vi "sv_Get Next Swept Frequency.vi"(7 "mode":enum16{"feedback", "deterministic"}(ring), 8 "error in (no error)":errorcluster, 11 "swept sine task in":T1={"source settings"={"AO task name"="", "source"=[]}, "stimulus settings"={"stimulus task name"="", "stimulus"=[]}, "response(s) settings"={"response task name"="", "response"=[]}, "measurement settings"={"AI sampling frequency"=51200.0, "AO sampling frequency"=1024.0, "AI block size"=1024, "AO block Size"=1024, "block duration [ms]"=1024.0, "number of AI channels"=0, "device propagation delay [samples]"=0.0, "total propagation time [samples]"=0.0, "DUT propagation time [ms]"=0.0}, "linlog"=enum."linear", "repeat"=enum."off", "frequency list"=[1.0], "amplitude list"=[1.0], "settling time"={"settle time"=0.015599999576807022, "settle cycles"=5}, "integration time"={"integration time"=0.015599999576807022, "integration cycles"=5}, "frequencies indices"={"AI freq index"=0, "AO freq index"=5}, "read marks"={"write index"=0, "read index"=0, "freq start index"=0, "freq stop index"=0, "# extracted"=0, "buffer type"=enum."Invalid buffer", "read/write indices"=[], "AO index"=0, "AI index"=0, "settled"=FALSE, "integration done"=FALSE}, "harmonic settings"={"maximum THD harmonic"=5, "harmonic mapping"=[1], "units"={"THD unit"=enum."%", "nth harmonic unit"=enum."%", "SINAD unit"=enum."dB", "THD+N unit"=enum."dB"}}, "auto resolution settings"={"auto max step"=512, "slow threshold db"=6.0, "fast threshold db"=1.0}, "auto level settings"={"auto level enable"=FALSE, "auto level channel"=6, "ideal ref"=1.0, "max level"=10.0, "ref upper deviation db"=3.0, "ref lower deviation db"=-3.0}, "offset"=1.0, "ramping rate"=0.0, "phase"=1.0, "initialize"=FALSE} {"phase" format="%.2f"; "response(s) settings"."response"."channel info"."pregain" format="%.2f"; "response(s) settings"."response"."channel info"."weighting filter" items=["Linear", "A-weighting", "B-weighting", "C-weighting", "ITU-R 468-4", "Dolby", "CCITT", "C-message", "Wb", "Wc", "Wd", "We", "Wf", "Wh", "Wj", "Wk", "Wm", "AES17 20 kHz lowpass", "AES17 40 kHz lowpass", "AES17 20 kHz highpass", "AES17 40 kHz highpass"]; "response(s) settings"."response"."channel info"."dB reference" format="%^.1e"; "response(s) settings"."response"."channel info"."engineering units" items=["custom..."=0, "V"=1, "A"=21, "C"=30, "pC"=31, "s"=32, "-"=29, "Pa"=2, "N"=20, "g"=3, "m/s^2"=4, "m/s"=5, "m"=6, "mm/s"=12, "mm"=13, "micron/s"=14, "micron"=15, "in/s^2"=7, "in/s"=8, "in"=9, "mil/s"=10, "mil"=11, "rad/s^2"=16, "rad/s"=17, "rad"=18, "deg/s^2"=26, "deg/s"=27, "deg"=28, "RPM"=22, "cycle/s^2"=23, "Hz"=24, "cycle"=25, "strain"=19]; "response(s) settings"."response"."channel info"."sensor sensitivity" format="%#_5f"; "stimulus settings"."stimulus"."channel info"."pregain" format="%.2f"; "stimulus settings"."stimulus"."channel info"."weighting filter" items=["Linear", "A-weighting", "B-weighting", "C-weighting", "ITU-R 468-4", "Dolby", "CCITT", "C-message", "Wb", "Wc", "Wd", "We", "Wf", "Wh", "Wj", "Wk", "Wm", "AES17 20 kHz lowpass", "AES17 40 kHz lowpass", "AES17 20 kHz highpass", "AES17 40 kHz highpass"]; "stimulus settings"."stimulus"."channel info"."dB reference" format="%^.1e"; "stimulus settings"."stimulus"."channel info"."engineering units" items=["custom..."=0, "V"=1, "A"=21, "C"=30, "pC"=31, "s"=32, "-"=29, "Pa"=2, "N"=20, "g"=3, "m/s^2"=4, "m/s"=5, "m"=6, "mm/s"=12, "mm"=13, "micron/s"=14, "micron"=15, "in/s^2"=7, "in/s"=8, "in"=9, "mil/s"=10, "mil"=11, "rad/s^2"=16, "rad/s"=17, "rad"=18, "deg/s^2"=26, "deg/s"=27, "deg"=28, "RPM"=22, "cycle/s^2"=23, "Hz"=24, "cycle"=25, "strain"=19]; "stimulus settings"."stimulus"."channel info"."sensor sensitivity" format="%#_5f"; "ramping rate" format="%.4f"; "offset" format="%.2f"; "auto level settings"."ref lower deviation db" format="%.4f"; "auto level settings"."ref upper deviation db" format="%.4f"; "auto level settings"."max level" format="%.4f"; "auto level settings"."ideal ref" format="%.4f"; "auto resolution settings"."fast threshold db" format="%.4f"; "auto resolution settings"."slow threshold db" format="%.4f"; "harmonic settings"."maximum THD harmonic" max=10 step=1; "integration time"."integration time" format="%.2p"; "settling time"."settle time" format="%.2p"; "amplitude list" format="%.2f"; "frequency list" format="%.2f"; "measurement settings"."DUT propagation time [ms]" format="%.2f"; "measurement settings"."AO sampling frequency" format="%.2f"; "measurement settings"."AI sampling frequency" format="%.2f"}) -> (0 "error out":errorcluster, 2 "stimulus":dbl[](array[numeric]) format="%.2f", 3 "swept sine task out":T1={"source settings"={"AO task name"="", "source"=[]}, "stimulus settings"={"stimulus task name"="", "stimulus"=[]}, "response(s) settings"={"response task name"="", "response"=[]}, "measurement settings"={"AI sampling frequency"=51200.0, "AO sampling frequency"=1024.0, "AI block size"=1024, "AO block Size"=1024, "block duration [ms]"=1024.0, "number of AI channels"=0, "device propagation delay [samples]"=0.0, "total propagation time [samples]"=0.0, "DUT propagation time [ms]"=0.0}, "linlog"=enum."linear", "repeat"=enum."off", "frequency list"=[1.0], "amplitude list"=[1.0], "settling time"={"settle time"=0.015599999576807022, "settle cycles"=5}, "integration time"={"integration time"=0.015599999576807022, "integration cycles"=5}, "frequencies indices"={"AI freq index"=0, "AO freq index"=5}, "read marks"={"write index"=0, "read index"=0, "freq start index"=0, "freq stop index"=0, "# extracted"=0, "buffer type"=enum."Invalid buffer", "read/write indices"=[], "AO index"=0, "AI index"=0, "settled"=FALSE, "integration done"=FALSE}, "harmonic settings"={"maximum THD harmonic"=5, "harmonic mapping"=[1], "units"={"THD unit"=enum."%", "nth harmonic unit"=enum."%", "SINAD unit"=enum."dB", "THD+N unit"=enum."dB"}}, "auto resolution settings"={"auto max step"=512, "slow threshold db"=6.0, "fast threshold db"=1.0}, "auto level settings"={"auto level enable"=FALSE, "auto level channel"=6, "ideal ref"=1.0, "max level"=10.0, "ref upper deviation db"=3.0, "ref lower deviation db"=-3.0}, "offset"=1.0, "ramping rate"=0.0, "phase"=1.0, "initialize"=FALSE} {"phase" format="%.2f"; "response(s) settings"."response"."channel info"."pregain" format="%.2f"; "response(s) settings"."response"."channel info"."weighting filter" items=["Linear", "A-weighting", "B-weighting", "C-weighting", "ITU-R 468-4", "Dolby", "CCITT", "C-message", "Wb", "Wc", "Wd", "We", "Wf", "Wh", "Wj", "Wk", "Wm", "AES17 20 kHz lowpass", "AES17 40 kHz lowpass", "AES17 20 kHz highpass", "AES17 40 kHz highpass"]; "response(s) settings"."response"."channel info"."dB reference" format="%^.1e"; "response(s) settings"."response"."channel info"."engineering units" items=["custom..."=0, "V"=1, "A"=21, "C"=30, "pC"=31, "s"=32, "-"=29, "Pa"=2, "N"=20, "g"=3, "m/s^2"=4, "m/s"=5, "m"=6, "mm/s"=12, "mm"=13, "micron/s"=14, "micron"=15, "in/s^2"=7, "in/s"=8, "in"=9, "mil/s"=10, "mil"=11, "rad/s^2"=16, "rad/s"=17, "rad"=18, "deg/s^2"=26, "deg/s"=27, "deg"=28, "RPM"=22, "cycle/s^2"=23, "Hz"=24, "cycle"=25, "strain"=19]; "response(s) settings"."response"."channel info"."sensor sensitivity" format="%#_5f"; "stimulus settings"."stimulus"."channel info"."pregain" format="%.2f"; "stimulus settings"."stimulus"."channel info"."weighting filter" items=["Linear", "A-weighting", "B-weighting", "C-weighting", "ITU-R 468-4", "Dolby", "CCITT", "C-message", "Wb", "Wc", "Wd", "We", "Wf", "Wh", "Wj", "Wk", "Wm", "AES17 20 kHz lowpass", "AES17 40 kHz lowpass", "AES17 20 kHz highpass", "AES17 40 kHz highpass"]; "stimulus settings"."stimulus"."channel info"."dB reference" format="%^.1e"; "stimulus settings"."stimulus"."channel info"."engineering units" items=["custom..."=0, "V"=1, "A"=21, "C"=30, "pC"=31, "s"=32, "-"=29, "Pa"=2, "N"=20, "g"=3, "m/s^2"=4, "m/s"=5, "m"=6, "mm/s"=12, "mm"=13, "micron/s"=14, "micron"=15, "in/s^2"=7, "in/s"=8, "in"=9, "mil/s"=10, "mil"=11, "rad/s^2"=16, "rad/s"=17, "rad"=18, "deg/s^2"=26, "deg/s"=27, "deg"=28, "RPM"=22, "cycle/s^2"=23, "Hz"=24, "cycle"=25, "strain"=19]; "stimulus settings"."stimulus"."channel info"."sensor sensitivity" format="%#_5f"; "ramping rate" format="%.4f"; "offset" format="%.2f"; "auto level settings"."ref lower deviation db" format="%.4f"; "auto level settings"."ref upper deviation db" format="%.4f"; "auto level settings"."max level" format="%.4f"; "auto level settings"."ideal ref" format="%.4f"; "auto resolution settings"."fast threshold db" format="%.4f"; "auto resolution settings"."slow threshold db" format="%.4f"; "harmonic settings"."maximum THD harmonic" max=10 step=1; "integration time"."integration time" format="%.2p"; "settling time"."settle time" format="%.2p"; "amplitude list" format="%.2f"; "frequency list" format="%.2f"; "measurement settings"."DUT propagation time [ms]" format="%.2f"; "measurement settings"."AO sampling frequency" format="%.2f"; "measurement settings"."AI sampling frequency" format="%.2f"}, 4 "current source frequency":dbl format="%.2f")   [LabVIEW 2017, in "SoundVib_SweptSine.lvlib"]
uses:
  <vilib>/addons/Sound and Vibration/svt_Swept Sine/SoundVib_SweptSine.lvlib
  <vilib>/addons/Sound and Vibration/svt_Swept Sine/subVIs/sv_Swept Sine Task.ctl
  <vilib>/addons/_NISVFA/_Shared subVIs/Controls/svc_Channel Info.ctl
  <vilib>/addons/_NISVFA/_Shared subVIs/Controls/svc_Engineering Units Text Ring.ctl
  <vilib>/addons/_NISVFA/_Shared subVIs/Controls/svc_Weighting Filter Text Ring.ctl
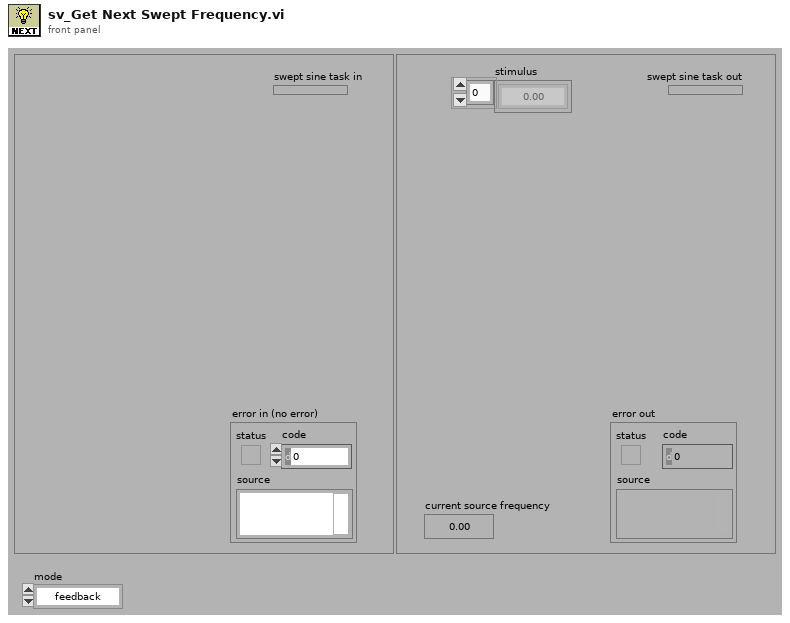
[diagram p1: front panel]
types:
  T1 = typedef "SoundVib_SweptSine.lvlib/sv_Swept Sine Task.ctl" = cluster{"source settings":cluster{"AO task name":refnum<k21>, "source":cluster{"AO physical channel":tag}[]}, "stimulus settings":cluster{"stimulus task name":refnum<k21>, "stimulus":cluster{"stimulus physical channel":tag, "channel info":T2}[]}, "response(s) settings":cluster{"response task name":refnum<k21>, "response":cluster{"response physical channel":tag, "channel info":T2}[]}, "measurement settings":cluster{"AI sampling frequency":dbl, "AO sampling frequency":dbl, "AI block size":i32, "AO block Size":i32, "block duration [ms]":dbl, "number of AI channels":i32, "device propagation delay [samples]":dbl, "total propagation time [samples]":dbl, "DUT propagation time [ms]":dbl}, "linlog":enum16{"linear", "log"}, "repeat":enum16{"off", "on"}, "frequency list":dbl[], "amplitude list":dbl[], "settling time":cluster{"settle time":dbl, "settle cycles":i32}, "integration time":cluster{"integration time":dbl, "integration cycles":i32}, "frequencies indices":cluster{"AI freq index":i32, "AO freq index":i32}, "read marks":cluster{"write index":u32, "read index":u32, "freq start index":u32, "freq stop index":u32, "# extracted":u32, "buffer type":enum16{"Invalid buffer", "Intermediate buffer", "Final buffer"}, "read/write indices":cluster{"settle time index":u32, "integration time index":u32}[], "AO index":i32, "AI index":i32, "settled":bool, "integration done":bool}, "harmonic settings":cluster{"maximum THD harmonic":u32, "harmonic mapping":u32[], "units":cluster{"THD unit":enum16{"dB", "%"}, "nth harmonic unit":enum16{"dB", "%"}, "SINAD unit":enum16{"dB", "%"}, "THD+N unit":enum16{"dB", "%"}}}, "auto resolution settings":cluster{"auto max step":i32, "slow threshold db":dbl, "fast threshold db":dbl}, "auto level settings":cluster{"auto level enable":bool, "auto level channel":u8, "ideal ref":sgl, "max level":sgl, "ref upper deviation db":sgl, "ref lower deviation db":sgl}, "offset":dbl, "ramping rate":dbl, "phase":dbl, "initialize":bool}
  T2 = typedef "svc_Channel Info.ctl" = cluster{"sensor sensitivity":dbl, "engineering units":T3, "dB reference":dbl, "custom label":string, "weighting filter":T4, "pregain":dbl}
  T3 = typedef "svc_Engineering Units Text Ring.ctl" = u16
  T4 = typedef "svc_Weighting Filter Text Ring.ctl" = u16
  T5 = enum16{"No Frequency Transition", "Transition to Next Frequency", "Transition to DC (last block)"}
  T6 = cluster{"freq start index":u32, "freq stop index":u32, "propagation time / 2":u32, "settle time samples":u32, "integration time samples":u32, "samples to zero crossing":u32, "non causal delay samples":u32, "end of block padding":u32}
  T7 = cluster{"integration time":dbl, "integration cycles":i32}
  T8 = cluster{"settle time index":u32, "integration time index":u32}[]
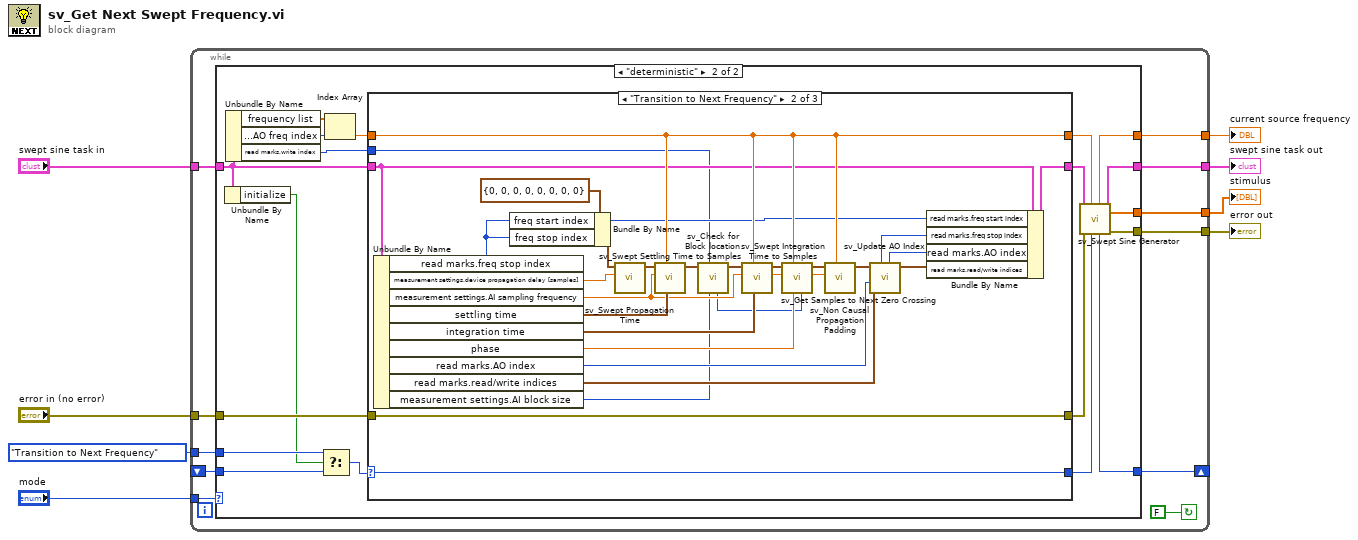
[diagram p0: block diagram]
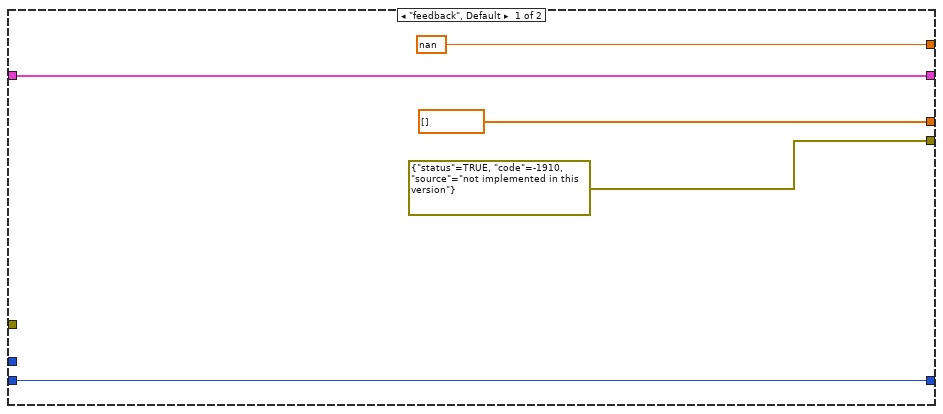
[diagram p2: hidden frame]
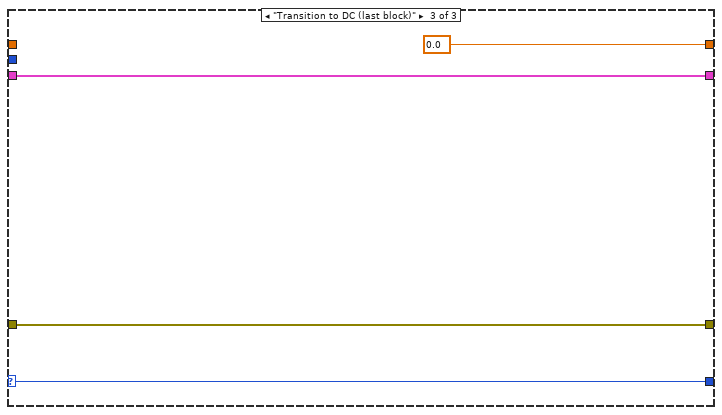
[diagram p4: hidden frame]
diagram:
  n1 = while {
    tunnel: "swept sine task in" -> [w15]
    tunnel: "error in (no error)" -> [w19]
    tunnel: "mode" -> [w18]
    shift-right: [w14] -> _
    shift-left: _ -> [w16]
    tunnel: [w13] -> w5
    tunnel: [w12] -> w4
    tunnel: [w11] -> w3
    tunnel: [w10] -> w2
    tunnel: T5."Transition to Next Frequency" ("t") -> [w9]
    stop <- FALSE continue-if-true
    n2 = case shown="\"deterministic\"" w18 {
      tunnel: [errorcluster {"status"=TRUE, "code"=-1910, "source"="not implemented in this version"} ("error in (no error)") w40] -> w12
      tunnel: [w24 w42] -> w13
      tunnel: w19 -> [_ w32]
      tunnel: w15 -> [w24 w26]
      tunnel: w16 -> [w22 w30]
      tunnel: [w22 w39] -> w14
      tunnel: [sgl[] [] ("Y") w38] -> w11
      tunnel: [nan ("t0") w37] -> w10
      tunnel: w9 -> [_ w29]
      frame "feedback", Default {
      }
      frame "deterministic" {
        n3 = Unbundle By Name(w26) -> ("initialize"=w25:bool)
        n4 = Unbundle By Name(w26) -> ("frequency list"=w35:dbl[], "frequencies indices.AO freq index"=w34:i32, "read marks.write index"=w27:u32)
        n5 = Select(t=w29, s=w25, f=w30) -> (s? t:f=w31:T5)
        n6 = Index Array(array=w35, index=w34) -> (element=w33:dbl)
        n7 = case shown="\"Transition to Next Frequency\"" w31 {
          selector: w31 -> [w45 w76 w78]
          tunnel: w26 -> [w47 w60 w79]
          tunnel: [w46 w67 w80] -> w41
          tunnel: [w47 w74 w79] -> w43
          tunnel: w32 -> [w46 w67 w80]
          tunnel: w33 -> [w44 w63 _]
          tunnel: [w45 w76 w78] -> w36
          tunnel: [w44 w63 0.0] -> w28
          tunnel: w27 -> [_ w49 _]
          frame "No Frequency Transition", Default {
          }
          frame "Transition to Next Frequency" {
            n8 = Unbundle By Name(w60) -> ("read marks.freq stop index"=w62:u32, "measurement settings.device propagation delay [samples]"=w72:dbl, "measurement settings.AI sampling frequency"=w54:dbl, "settling time"=w70:cluster{"settle time":dbl, "settle cycles":i32}, "integration time"=w59:T7, "phase"=w75:dbl, "read marks.AO index"=w57:i32, "read marks.read/write indices"=w58:T8, "measurement settings.AI block size"=w50:i32)
            n9 = Bundle By Name(cluster=T6 {"freq start index"=0, "freq stop index"=0, "propagation time / 2"=0, "settle time samples"=0, "integration time samples"=0, "samples to zero crossing"=0, "non causal delay samples"=0, "end of block padding"=0} ("indice computations in"), "freq start index"=w62, "freq stop index"=w62) -> (w61:T6)
            n10 = call <vilib>:"sv_Swept Propagation Time.vi"("board propagation time [samples]"=w72, "indice computations in"=w61) -> ("indice computations in"=w71:T6)  [unwired: 9 in]
            n11 = call <vilib>:"sv_Swept Settling Time to Samples.vi"("settling time"=w70, "frequency to generate [Hz]"=w63, "AI sampling frequency"=w54, "indice computations in"=w71) -> ("indice computations in"=w56:T6)  [unwired: 6 in, 1 out]
            n12 = call <vilib>:"sv_Check for Block location.vi"("AI block size"=w50, "write index"=w49, "indice computations in"=w56) -> ("indice computations in"=w55:T6, "write index - block size"=w48:u32)  [unwired: 7 in]
            n13 = call <vilib>:"sv_Swept Integration Time to Samples.vi"("integration time"=w59, "frequency to generate [Hz]"=w63, "AI sampling frequency"=w54, "indice computations in"=w55) -> ("dup AI sampling frequency"=w52:dbl, "indice computations in"=w53:T6)  [unwired: 6 in]
            n14 = call <vilib>:"sv_Get Samples to Next Zero Crossing .vi"("write index - block size"=w48, "phase"=w75, "frequency to generate [Hz]"=w63, "AI sampling frequency"=w52, "indice computations in"=w53) -> ("dup AI sampling frequency"=w68:dbl, "indice computations in"=w69:T6)  [unwired: 5 in]
            n15 = call <vilib>:"sv_Non Causal Propagation Padding .vi"("frequency to generate [Hz]"=w63, "AI sampling frequency"=w68, "indice computations in"=w69) -> ("indice computations in"=w51:T6)  [unwired: 8 in]
            n16 = call <vilib>:"sv_Update AO Index.vi"("read/write indices"=w58, "current AO index"=w57, "indice computations in"=w51) -> ("new read/write indices"=w64:T8, "new AO index"=w65:i32, "new freq stop index"=w66:u32)  [unwired: 6 in]
            n17 = Bundle By Name(cluster=w60, "read marks.freq start index"=w62, "read marks.freq stop index"=w66, "read marks.AO index"=w65, "read marks.read/write indices"=w64) -> (w74:T1)
          }
          frame "Transition to DC (last block)" {
          }
        }
        n18 = call <vilib>:"sv_Swept Sine Generator.vi"("case in"=w36, "frequency to generate [Hz]"=w28, "error in (no error)"=w41, "swept sine task in"=w43) -> ("error out"=w40:errorcluster, "stimulus"=w38:dbl[], "swept sine task out"=w42:T1, "case"=w39:T5, "dup frequency to generate [Hz]"=w37:dbl)  [unwired: 3 in]
      }
    }
  }
  "current source frequency" <- w2
  "error out" <- w4
  "swept sine task out" <- w5
  "stimulus" <- w3
